vi "Launch Nested Actor.vi"(4 "Debug Alias":string, 6 "Open Actor Core front panel? (F)":bool, 8 "error in (no error)":errorcluster, 9 "Auto-stop? (T)":bool=TRUE, 10 "Nested Actor":refnum<class "Actor.lvclass">, 11 "Caller Actor in":refnum<class "Actor.lvclass">) -> (0 "error out":errorcluster, 2 "Nested Actor's Enqueuer":refnum<class "Message Enqueuer.lvclass">, 3 "Caller Actor out":refnum<class "Actor.lvclass">)   [LabVIEW 2020, in "Actor Framework.lvlib" / "Actor.lvclass"]
doc: "<p>(<strong>Filename</strong>: <span class=\"dnl\">Actor Framework.lvlib:Actor.lvclass:Launch Nested Actor.vi</span>)</p>\n\n<p>Launches an asynchronously running VI that performs tasks and handles messages for the <strong>Nested Actor</strong>. Use this VI to launch actors that are dependent on one or more calling actors. This VI returns a reference to the enqueuer that you can use to send messages to the newly launched actor.</p>\n\n<p>This VI requires the <strong>Caller Actor in</strong> input to call the <strong>Nested Actor</strong>. This VI will return an error if the <strong>Caller Actor in</strong> has not already been launched itself. Use the <a href=\"nihelplauncher://docs/csh?context=lvcore_lvcomm_af_launch_root_actor\">Launch Root Actor VI</a> for launching an actor without a caller.</p>"
uses:
  Actor.lvclass
  Message Enqueuer/Message Enqueuer.lvclass
  Actor.lvclass/Actor.ctl
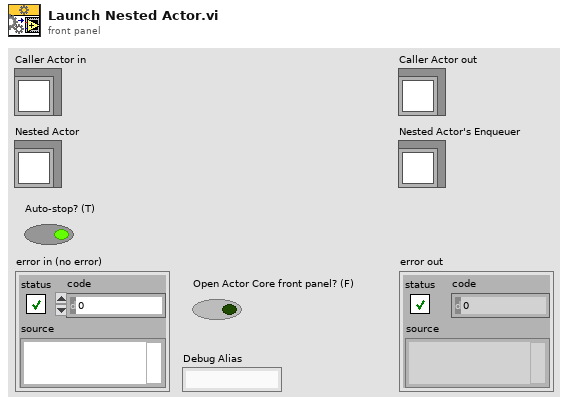
[diagram p1: front panel]
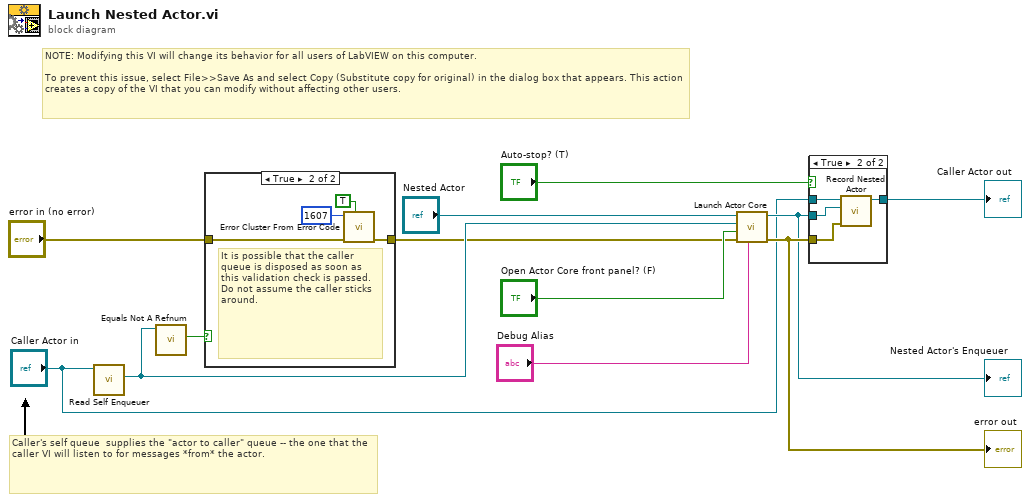
[diagram p0: block diagram]
diagram:
  # "Caller's self queue  supplies the \"actor to caller\" queue -- the one that the caller VI will listen to for messages *from* the actor."
  # "NOTE: Modifying this VI will change its behavior for all users of LabVIEW on this computer.\n\nTo prevent this issue, select File>>Save As and select Copy (Substitute copy for original) in the dialog box that appears. This action creates a copy of the VI that you can modify without affecting other users."
  n1 = call "Read Self Enqueuer.vi"("Actor"="Caller Actor in") -> ("Self Enqueuer"=w11:refnum<class "Message Enqueuer.lvclass">)  [unwired: 10 in]
  n2 = call "Equals Not A Refnum.vi"("Message Enqueuer"=w11) -> ("Not a refnum?"=w10:bool)  [unwired: 10 in]
  n3 = case shown="True" w10 {
    tunnel: "error in (no error)" -> [w13 w17]
    tunnel: [w13 w16] -> w2
    frame False {
    }
    frame True {
      # "It is possible that the caller queue is disposed as soon as this validation check is passed. Do not assume the caller sticks around."
      n4 = call <vilib>:"Error Cluster From Error Code.vi"("show call chain? (False)"=TRUE, "error in (no error)"=w17, "error code (0)"=1607) -> ("error out"=w16:errorcluster)  [unwired: 6 in]
    }
  }
  n5 = call "Launch Actor Core.vi"("Debug Alias"="Debug Alias", "error in (no error)"=w2, "Open Actor Core front panel?"="Open Actor Core front panel? (F)", "Caller's Enqueuer"=w11, "Actor in"="Nested Actor") -> ("error out"=w6:errorcluster, "Message Enqueuer out"=w4:refnum<class "Message Enqueuer.lvclass">)  [unwired: 5 in]
  "error out" <- w6
  "Nested Actor's Enqueuer" <- w4
  n6 = case shown="True" "Auto-stop? (T)" {
    tunnel: "Caller Actor in" -> [w18 w22]
    tunnel: [w18 w21] -> w7
    tunnel: w6 -> [_ w20]
    tunnel: w4 -> [_ w19]
    frame False {
    }
    frame True {
      n7 = call "Record Nested Actor.vi"("error in (no error)"=w20, "Message Enqueuer"=w19, "Actor in"=w22) -> ("Actor out"=w21:refnum<class "Actor.lvclass">)  [unwired: 8 in]
    }
  }
  "Caller Actor out" <- w7
